vi "Handle GOODBYE.vi"(9 "WAMP Message":T1 {"Message Codes" items=["HELLO"=1, "WELCOME"=2, "ABORT"=3, "GOODBYE"=6, "ERROR"=8, "PUBLISH"=16, "PUBLISHED"=17, "SUBSCRIBE"=32, "SUBSCRIBED"=33, "UNSUBSCRIBE"=34, "UNSUBSCRIBED"=35, "EVENT"=36, "CALL"=48, "RESULT"=59, "REGISTER"=64, "REGISTERED"=65, "UNREGISTER"=66, "UNREGISTERED"=67, "INVOCATION"=68, "YIELD"=70]}, 10 "error in (no error)":errorcluster, 11 "WAMP Client in":refnum<class "WAMP Client.lvclass">) -> (2 "error out":errorcluster, 3 "WAMP Client out":refnum<class "WAMP Client.lvclass">)   [LabVIEW 2020]
uses:
  <userlib>/wamplv/WAMP Client/WAMP Client.lvclass
  <userlib>/wamplv/WAMP Message Codes.ctl
  <userlib>/wamplv/WAMP Client/TypeDef/WAMP Received Message.ctl
panel:
  out "element":string
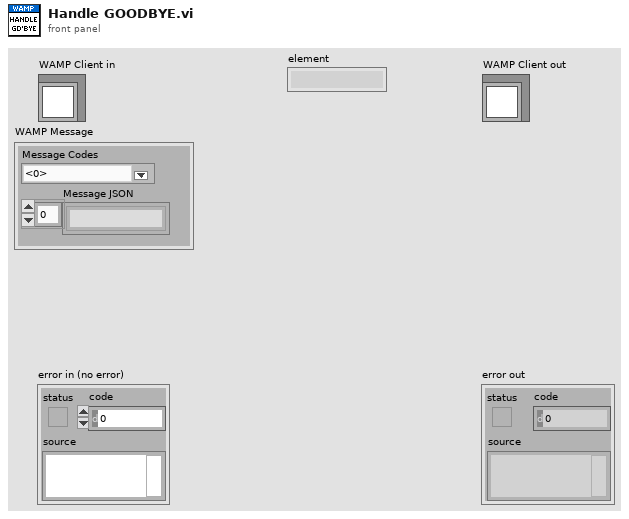
[diagram p1: front panel]
types:
  T1 = typedef "wamplv.lvlib/WAMP Client.lvclass/WAMP Received Message.ctl" = cluster{"Message JSON":string[], "Message Codes":T2}
  T2 = typedef "wamplv.lvlib/WAMP Client.lvclass/WAMP Message Codes.ctl" = u16
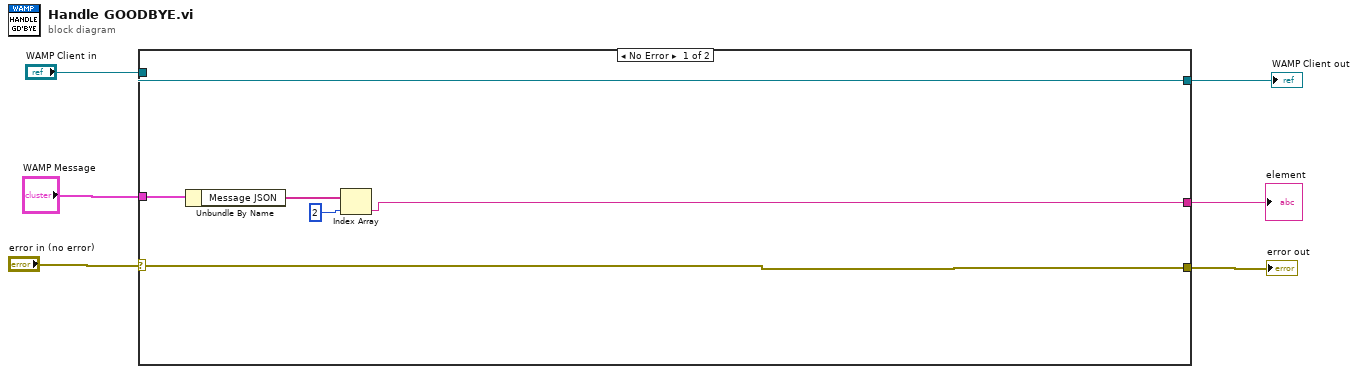
[diagram p0: block diagram]
diagram:
  n1 = case shown="No Error" "error in (no error)" {
    selector: "error in (no error)" -> [w8 w14]
    tunnel: [w8 w14] -> w5
    tunnel: [w12 w13] -> w3
    tunnel: "WAMP Client in" -> [w12 w13]
    tunnel: "WAMP Message" -> [w11 _]
    tunnel: [w7 _] -> w1
    frame No Error {
      n2 = Unbundle By Name(w11) -> ("Message JSON"=w10:string[])
      n3 = Index Array(array=w10, index=2) -> (element=w7:string)
    }
    frame Error {
    }
  }
  "error out" <- w5
  "WAMP Client out" <- w3
  "element" <- w1
